vi "Lab Panel V5.23.vi"() -> ()   [LabVIEW 2013] (continued)
                          }
                        }
                        n2194 = local read "Panel #"() -> (w3891:dbl)
                        n2195 = case shown="1" w3891 {
                          tunnel: w3892 -> [_ w3899]
                          tunnel: w3889 -> [_ w3898]
                          frame 0, Default {
                          }
                          frame 1 {
                            n2196 = Multiply(x=w3899, y=w3898) -> (x*y=w3897:dbl)
                            n2197 = Subtract(x=w3897, y=272) -> (x-y=w3895:dbl)
                            "Amb Tp" <- w3895
                            n2198 = local write "Ref deg C"(w3895) -> ()
                          }
                        }
                        "deg C (volts)" <- w3889
                      }
                      frame True {
                      }
                    }
                  }
                }
              }
            }
          }
          frame #12 {
            # "save test data to file"
            n2199 = Get Date/Time In Seconds() -> (seconds since 1Jan1904=w3900:timestamp)
            "File Time Stamp" <- w3900
            n2200 = local read "on loops"() -> (w3919:dbl)
            n2201 = local read "jig cycle"() -> (w3916:dbl)
            n2202 = Format Date/Time String(time format string (%c)="%H:%M%:%S", seconds (now)=w3900) -> (date/time string=w3904:string)  [unwired: 1 in]
            n2203 = Add(x=w3919, y=2) -> (x+y=w3917:dbl)
            n2204 = Build Array(w3904) -> (w3903:string[])
            n2205 = Equal?(x=w3916, y=1) -> (x = y?=w3902:bool)
            n2206 = Equal?(x=w3916, y=w3917) -> (x = y?=w3901:bool)
            n2207 = stacked-sequence {
              tunnel: w3915 -> [w3925 _ _ _ _ _ _ _ _ _]
              tunnel: w3914 -> [_ w4001 _ _ _ _ _ _ _ _]
              tunnel: w3913 -> [_ _ w4081 _ _ _ _ _ _ _]
              tunnel: w3912 -> [_ _ _ w4161 _ _ _ _ _ _]
              tunnel: w3911 -> [_ _ _ _ w4241 _ _ _ _ _]
              tunnel: w3910 -> [_ _ _ _ _ w4321 _ _ _ _]
              tunnel: w3909 -> [_ _ _ _ _ _ w4401 _ _ _]
              tunnel: w3908 -> [_ _ _ _ _ _ _ w4481 _ _]
              tunnel: w3907 -> [_ _ _ _ _ _ _ _ w4561 _]
              tunnel: w3906 -> [_ _ _ _ _ _ _ _ _ w4641]
              tunnel: w3903 -> [w3924 w4005 w4085 w4165 w4245 w4325 w4405 w4485 w4565 w4645]
              tunnel: w3902 -> [w3923 w4004 w4084 w4164 w4244 w4324 w4404 w4484 w4564 w4644]
              tunnel: w3901 -> [w3922 w4003 w4083 w4163 w4243 w4323 w4403 w4483 w4563 w4643]
              tunnel: w3900 -> [w3921 w4002 w4082 w4162 w4242 w4322 w4402 w4482 w4562 w4642]
              frame #0 {
                n2208 = case shown="True" w3925 {
                  tunnel: w3924 -> [_ w3930]
                  tunnel: w3923 -> [_ w3929]
                  tunnel: w3922 -> [_ w3927]
                  tunnel: w3921 -> [_ w3926]
                  frame False {
                  }
                  frame True {
                    n2209 = local read "DISP LAB01-1"() -> (w3931:T4)
                    n2210 = local read "SIG LAB01-1"() -> (w3932:T2)
                    n2211 = local read "ON L01-1"() -> (w3928:cluster{"amps":dbl, "volts":dbl, "pf":dbl})
                    n2212 = Unbundle(w3932) -> ("AMPS"=w3938:dbl, "VOLTS"=w3936:dbl, "PF"=w3935:dbl, "Tmp Live"=w3934:dbl, "Tmp Neut"=w3937:dbl)
                    n2213 = Unbundle(w3931) -> ("CYCLE"=w3933:dbl)  [unwired: 2 out]
                    n2214 = stacked-sequence {
                      tunnel: w3938 -> [w3942 w3961]
                      tunnel: w3937 -> [_ w3960]
                      tunnel: w3936 -> [w3941 w3959]
                      tunnel: w3935 -> [w3940 w3958]
                      tunnel: w3934 -> [_ w3957]
                      tunnel: w3933 -> [_ w3956]
                      tunnel: w3930 -> [_ w3955]
                      tunnel: w3929 -> [w3943 _]
                      tunnel: w3928 -> [w3939 w3953]
                      tunnel: w3927 -> [_ w3954]
                      tunnel: w3926 -> [_ w3949]
                      frame #0 {
                        n2215 = case shown="True" w3943 {
                          tunnel: w3942 -> [_ w3948]
                          tunnel: w3941 -> [_ w3947]
                          tunnel: w3940 -> [_ w3946]
                          tunnel: w3939 -> [_ w3944]
                          frame False {
                          }
                          frame True {
                            n2216 = Bundle(cluster=w3944, "amps"=w3948, "volts"=w3947, "pf"=w3946) -> (w3945:cluster{"amps":dbl, "volts":dbl, "pf":dbl})
                            n2217 = local write "ON L01-1"(w3945) -> ()
                          }
                        }
                      }
                      frame #1 {
                        n2218 = Unbundle(w3953) -> ("amps"=w3952:dbl, "volts"=w3951:dbl, "pf"=w3950:dbl)
                        n2219 = case shown="True" w3954 {
                          tunnel: w3961 -> [_ w3962]
                          tunnel: w3960 -> [_ w4000]
                          tunnel: w3959 -> [_ _]
                          tunnel: w3958 -> [_ _]
                          tunnel: w3957 -> [_ w3999]
                          tunnel: w3956 -> [_ w3998]
                          tunnel: w3955 -> [_ w3966]
                          tunnel: w3952 -> [_ w3963]
                          tunnel: w3951 -> [_ w3995]
                          tunnel: w3950 -> [_ w3994]
                          tunnel: w3949 -> [_ w3964]
                          frame False {
                          }
                          frame True {
                            n2220 = local read "TDMS LAB01-1"() -> (w3997:refnum<k34>)
                            n2221 = Build Array(w3995) -> (w3991:dbl[])
                            n2222 = Build Array(w3994) -> (w3990:dbl[])
                            n2223 = Build Array(w3999) -> (w3989:dbl[])
                            n2224 = Build Array(w4000) -> (w3988:dbl[])
                            n2225 = Build Array(w3963) -> (w3993:dbl[])
                            n2226 = Build Array(w3962) -> (w3992:dbl[])
                            n2227 = Build Array(w3998) -> (w3987:dbl[])
                            n2228 = Build Array("AMPS ON", "AMPS OFF", "VOLTS", "PF", "TEMP Live", "TEMP Neut", "CYCLE") -> (w3971:string[])
                            n2229 = Bundle By Name("Y"=w3993, "t0"=w3964) -> (w3986:waveform(dbl))  [unwired: 1 in]
                            n2230 = Bundle By Name("Y"=w3992, "t0"=w3964) -> (w3985:waveform(dbl))  [unwired: 1 in]
                            n2231 = Bundle By Name("Y"=w3991, "t0"=w3964) -> (w3984:waveform(dbl))  [unwired: 1 in]
                            n2232 = Bundle By Name("Y"=w3990, "t0"=w3964) -> (w3983:waveform(dbl))  [unwired: 1 in]
                            n2233 = Bundle By Name("Y"=w3989, "t0"=w3964) -> (w3982:waveform(dbl))  [unwired: 1 in]
                            n2234 = Bundle By Name("Y"=w3988, "t0"=w3964) -> (w3981:waveform(dbl))  [unwired: 1 in]
                            n2235 = Bundle By Name("Y"=w3987, "t0"=w3964) -> (w3980:waveform(dbl))  [unwired: 1 in]
                            n2236 = Build Array(w3986, w3985, w3984, w3983, w3982, w3981, w3980) -> (w3979:waveform(dbl)[])
                            n2237 = TDMS Write(0:w3997, 5:"TEST VALUES", 7:w3971, 9:w3979) -> (4:w3970:refnum<k34>, 6:w3969:string, 15:w3968:errorcluster)  [unwired: 2 in, 1 out]
                            n2238 = TDMS Write(0:w3970, 5:w3969, 7:"TIME", 9:w3966, 11:w3968) -> (15:w3965:errorcluster)  [unwired: 1 in, 3 out]
                            n2239 = local write "data file error"(w3965) -> ()
                          }
                        }
                      }
                    }
                  }
                }
              }
              frame #1 {
                n2240 = case shown="True" w4001 {
                  tunnel: w4005 -> [_ w4010]
                  tunnel: w4004 -> [_ w4009]
                  tunnel: w4003 -> [_ w4007]
                  tunnel: w4002 -> [_ w4006]
                  frame False {
                  }
                  frame True {
                    n2241 = local read "DISP LAB01-2"() -> (w4011:T4)
                    n2242 = local read "SIG LAB01-2"() -> (w4012:T2)
                    n2243 = local read "ON L01-2"() -> (w4008:cluster{"amps":dbl, "volts":dbl, "pf":dbl})
                    n2244 = Unbundle(w4012) -> ("AMPS"=w4018:dbl, "VOLTS"=w4016:dbl, "PF"=w4015:dbl, "Tmp Live"=w4014:dbl, "Tmp Neut"=w4017:dbl)
                    n2245 = Unbundle(w4011) -> ("CYCLE"=w4013:dbl)  [unwired: 2 out]
                    n2246 = stacked-sequence {
                      tunnel: w4018 -> [w4022 w4041]
                      tunnel: w4017 -> [_ w4040]
                      tunnel: w4016 -> [w4021 w4039]
                      tunnel: w4015 -> [w4020 w4038]
                      tunnel: w4014 -> [_ w4037]
                      tunnel: w4013 -> [_ w4036]
                      tunnel: w4010 -> [_ w4035]
                      tunnel: w4009 -> [w4023 _]
                      tunnel: w4008 -> [w4019 w4033]
                      tunnel: w4007 -> [_ w4034]
                      tunnel: w4006 -> [_ w4029]
                      frame #0 {
                        n2247 = case shown="True" w4023 {
                          tunnel: w4022 -> [_ w4028]
                          tunnel: w4021 -> [_ w4027]
                          tunnel: w4020 -> [_ w4026]
                          tunnel: w4019 -> [_ w4024]
                          frame False {
                          }
                          frame True {
                            n2248 = Bundle(cluster=w4024, "amps"=w4028, "volts"=w4027, "pf"=w4026) -> (w4025:cluster{"amps":dbl, "volts":dbl, "pf":dbl})
                            n2249 = local write "ON L01-2"(w4025) -> ()
                          }
                        }
                      }
                      frame #1 {
                        n2250 = Unbundle(w4033) -> ("amps"=w4032:dbl, "volts"=w4031:dbl, "pf"=w4030:dbl)
                        n2251 = case shown="True" w4034 {
                          tunnel: w4041 -> [_ w4073]
                          tunnel: w4040 -> [_ w4080]
                          tunnel: w4039 -> [_ _]
                          tunnel: w4038 -> [_ _]
                          tunnel: w4037 -> [_ w4079]
                          tunnel: w4036 -> [_ w4078]
                          tunnel: w4035 -> [_ w4043]
                          tunnel: w4032 -> [_ w4075]
                          tunnel: w4031 -> [_ w4074]
                          tunnel: w4030 -> [_ w4072]
                          tunnel: w4029 -> [_ w4064]
                          frame False {
                          }
                          frame True {
                            n2252 = local read "TDMS LAB01-2"() -> (w4077:refnum<k34>)
                            n2253 = Build Array(w4074) -> (w4069:dbl[])
                            n2254 = Build Array(w4072) -> (w4068:dbl[])
                            n2255 = Build Array(w4079) -> (w4067:dbl[])
                            n2256 = Build Array(w4080) -> (w4066:dbl[])
                            n2257 = Build Array(w4075) -> (w4071:dbl[])
                            n2258 = Build Array(w4073) -> (w4070:dbl[])
                            n2259 = Build Array(w4078) -> (w4065:dbl[])
                            n2260 = Build Array("AMPS ON", "AMPS OFF", "VOLTS", "PF", "TEMP Live", "TEMP Neut", "CYCLE") -> (w4048:string[])
                            n2261 = Bundle By Name("Y"=w4071, "t0"=w4064) -> (w4063:waveform(dbl))  [unwired: 1 in]
                            n2262 = Bundle By Name("Y"=w4070, "t0"=w4064) -> (w4062:waveform(dbl))  [unwired: 1 in]
                            n2263 = Bundle By Name("Y"=w4069, "t0"=w4064) -> (w4061:waveform(dbl))  [unwired: 1 in]
                            n2264 = Bundle By Name("Y"=w4068, "t0"=w4064) -> (w4060:waveform(dbl))  [unwired: 1 in]
                            n2265 = Bundle By Name("Y"=w4067, "t0"=w4064) -> (w4059:waveform(dbl))  [unwired: 1 in]
                            n2266 = Bundle By Name("Y"=w4066, "t0"=w4064) -> (w4058:waveform(dbl))  [unwired: 1 in]
                            n2267 = Bundle By Name("Y"=w4065, "t0"=w4064) -> (w4057:waveform(dbl))  [unwired: 1 in]
                            n2268 = Build Array(w4063, w4062, w4061, w4060, w4059, w4058, w4057) -> (w4056:waveform(dbl)[])
                            n2269 = TDMS Write(0:w4077, 5:"TEST VALUES", 7:w4048, 9:w4056) -> (4:w4047:refnum<k34>, 6:w4046:string, 15:w4045:errorcluster)  [unwired: 2 in, 1 out]
                            n2270 = TDMS Write(0:w4047, 5:w4046, 7:"TIME", 9:w4043, 11:w4045) -> (15:w4042:errorcluster)  [unwired: 1 in, 3 out]
                            n2271 = local write "data file error"(w4042) -> ()
                          }
                        }
                      }
                    }
                  }
                }
              }
              frame #2 {
                n2272 = case shown="True" w4081 {
                  tunnel: w4085 -> [_ w4090]
                  tunnel: w4084 -> [_ w4089]
                  tunnel: w4083 -> [_ w4087]
                  tunnel: w4082 -> [_ w4086]
                  frame False {
                  }
                  frame True {
                    n2273 = local read "DISP LAB02-1"() -> (w4091:T4)
                    n2274 = local read "SIG LAB02-1"() -> (w4092:T2)
                    n2275 = local read "ON L02-1"() -> (w4088:cluster{"amps":dbl, "volts":dbl, "pf":dbl})
                    n2276 = Unbundle(w4092) -> ("AMPS"=w4098:dbl, "VOLTS"=w4096:dbl, "PF"=w4095:dbl, "Tmp Live"=w4094:dbl, "Tmp Neut"=w4097:dbl)
                    n2277 = Unbundle(w4091) -> ("CYCLE"=w4093:dbl)  [unwired: 2 out]
                    n2278 = stacked-sequence {
                      tunnel: w4098 -> [w4102 w4121]
                      tunnel: w4097 -> [_ w4120]
                      tunnel: w4096 -> [w4101 w4119]
                      tunnel: w4095 -> [w4100 w4118]
                      tunnel: w4094 -> [_ w4117]
                      tunnel: w4093 -> [_ w4116]
                      tunnel: w4090 -> [_ w4115]
                      tunnel: w4089 -> [w4103 _]
                      tunnel: w4088 -> [w4099 w4113]
                      tunnel: w4087 -> [_ w4114]
                      tunnel: w4086 -> [_ w4109]
                      frame #0 {
                        n2279 = case shown="True" w4103 {
                          tunnel: w4102 -> [_ w4108]
                          tunnel: w4101 -> [_ w4107]
                          tunnel: w4100 -> [_ w4106]
                          tunnel: w4099 -> [_ w4104]
                          frame False {
                          }
                          frame True {
                            n2280 = Bundle(cluster=w4104, "amps"=w4108, "volts"=w4107, "pf"=w4106) -> (w4105:cluster{"amps":dbl, "volts":dbl, "pf":dbl})
                            n2281 = local write "ON L02-1"(w4105) -> ()
                          }
                        }
                      }
                      frame #1 {
                        n2282 = Unbundle(w4113) -> ("amps"=w4112:dbl, "volts"=w4111:dbl, "pf"=w4110:dbl)
                        n2283 = case shown="True" w4114 {
                          tunnel: w4121 -> [_ w4153]
                          tunnel: w4120 -> [_ w4160]
                          tunnel: w4119 -> [_ _]
                          tunnel: w4118 -> [_ _]
                          tunnel: w4117 -> [_ w4159]
                          tunnel: w4116 -> [_ w4158]
                          tunnel: w4115 -> [_ w4123]
                          tunnel: w4112 -> [_ w4155]
                          tunnel: w4111 -> [_ w4154]
                          tunnel: w4110 -> [_ w4152]
                          tunnel: w4109 -> [_ w4144]
                          frame False {
                          }
                          frame True {
                            n2284 = local read "TDMS LAB02-1"() -> (w4157:refnum<k34>)
                            n2285 = Build Array(w4154) -> (w4149:dbl[])
                            n2286 = Build Array(w4152) -> (w4148:dbl[])
                            n2287 = Build Array(w4159) -> (w4147:dbl[])
                            n2288 = Build Array(w4160) -> (w4146:dbl[])
                            n2289 = Build Array(w4155) -> (w4151:dbl[])
                            n2290 = Build Array(w4153) -> (w4150:dbl[])
                            n2291 = Build Array(w4158) -> (w4145:dbl[])
                            n2292 = Build Array("AMPS ON", "AMPS OFF", "VOLTS", "PF", "TEMP Live", "TEMP Neut", "CYCLE") -> (w4128:string[])
                            n2293 = Bundle By Name("Y"=w4151, "t0"=w4144) -> (w4143:waveform(dbl))  [unwired: 1 in]
                            n2294 = Bundle By Name("Y"=w4150, "t0"=w4144) -> (w4142:waveform(dbl))  [unwired: 1 in]
                            n2295 = Bundle By Name("Y"=w4149, "t0"=w4144) -> (w4141:waveform(dbl))  [unwired: 1 in]
                            n2296 = Bundle By Name("Y"=w4148, "t0"=w4144) -> (w4140:waveform(dbl))  [unwired: 1 in]
                            n2297 = Bundle By Name("Y"=w4147, "t0"=w4144) -> (w4139:waveform(dbl))  [unwired: 1 in]
                            n2298 = Bundle By Name("Y"=w4146, "t0"=w4144) -> (w4138:waveform(dbl))  [unwired: 1 in]
                            n2299 = Bundle By Name("Y"=w4145, "t0"=w4144) -> (w4137:waveform(dbl))  [unwired: 1 in]
                            n2300 = Build Array(w4143, w4142, w4141, w4140, w4139, w4138, w4137) -> (w4136:waveform(dbl)[])
                            n2301 = TDMS Write(0:w4157, 5:"TEST VALUES", 7:w4128, 9:w4136) -> (4:w4127:refnum<k34>, 6:w4126:string, 15:w4125:errorcluster)  [unwired: 2 in, 1 out]
                            n2302 = TDMS Write(0:w4127, 5:w4126, 7:"TIME", 9:w4123, 11:w4125) -> (15:w4122:errorcluster)  [unwired: 1 in, 3 out]
                            n2303 = local write "data file error"(w4122) -> ()
                          }
                        }
                      }
                    }
                  }
                }
              }
              frame #3 {
                n2304 = case shown="True" w4161 {
                  tunnel: w4165 -> [_ w4170]
                  tunnel: w4164 -> [_ w4169]
                  tunnel: w4163 -> [_ w4167]
                  tunnel: w4162 -> [_ w4166]
                  frame False {
                  }
                  frame True {
                    n2305 = local read "DISP LAB02-2"() -> (w4171:T4)
                    n2306 = local read "SIG LAB02-2"() -> (w4172:T2)
                    n2307 = local read "ON L02-2"() -> (w4168:cluster{"amps":dbl, "volts":dbl, "pf":dbl})
                    n2308 = Unbundle(w4172) -> ("AMPS"=w4178:dbl, "VOLTS"=w4176:dbl, "PF"=w4175:dbl, "Tmp Live"=w4174:dbl, "Tmp Neut"=w4177:dbl)
                    n2309 = Unbundle(w4171) -> ("CYCLE"=w4173:dbl)  [unwired: 2 out]
                    n2310 = stacked-sequence {
                      tunnel: w4178 -> [w4182 w4201]
                      tunnel: w4177 -> [_ w4200]
                      tunnel: w4176 -> [w4181 w4199]
                      tunnel: w4175 -> [w4180 w4198]
                      tunnel: w4174 -> [_ w4197]
                      tunnel: w4173 -> [_ w4196]
                      tunnel: w4170 -> [_ w4195]
                      tunnel: w4169 -> [w4183 _]
                      tunnel: w4168 -> [w4179 w4193]
                      tunnel: w4167 -> [_ w4194]
                      tunnel: w4166 -> [_ w4189]
                      frame #0 {
                        n2311 = case shown="True" w4183 {
                          tunnel: w4182 -> [_ w4188]
                          tunnel: w4181 -> [_ w4187]
                          tunnel: w4180 -> [_ w4186]
                          tunnel: w4179 -> [_ w4184]
                          frame False {
                          }
                          frame True {
                            n2312 = Bundle(cluster=w4184, "amps"=w4188, "volts"=w4187, "pf"=w4186) -> (w4185:cluster{"amps":dbl, "volts":dbl, "pf":dbl})
                            n2313 = local write "ON L02-2"(w4185) -> ()
                          }
                        }
                      }
                      frame #1 {
                        n2314 = Unbundle(w4193) -> ("amps"=w4192:dbl, "volts"=w4191:dbl, "pf"=w4190:dbl)
                        n2315 = case shown="True" w4194 {
                          tunnel: w4201 -> [_ w4233]
                          tunnel: w4200 -> [_ w4240]
                          tunnel: w4199 -> [_ _]
                          tunnel: w4198 -> [_ _]
                          tunnel: w4197 -> [_ w4239]
                          tunnel: w4196 -> [_ w4238]
                          tunnel: w4195 -> [_ w4203]
                          tunnel: w4192 -> [_ w4235]
                          tunnel: w4191 -> [_ w4234]
                          tunnel: w4190 -> [_ w4232]
                          tunnel: w4189 -> [_ w4224]
                          frame False {
                          }
                          frame True {
                            n2316 = local read "TDMS LAB02-2"() -> (w4237:refnum<k34>)
                            n2317 = Build Array(w4234) -> (w4229:dbl[])
                            n2318 = Build Array(w4232) -> (w4228:dbl[])
                            n2319 = Build Array(w4239) -> (w4227:dbl[])
                            n2320 = Build Array(w4240) -> (w4226:dbl[])
                            n2321 = Build Array(w4235) -> (w4231:dbl[])
                            n2322 = Build Array(w4233) -> (w4230:dbl[])
                            n2323 = Build Array(w4238) -> (w4225:dbl[])
                            n2324 = Build Array("AMPS ON", "AMPS OFF", "VOLTS", "PF", "TEMP Live", "TEMP Neut", "CYCLE") -> (w4208:string[])
                            n2325 = Bundle By Name("Y"=w4231, "t0"=w4224) -> (w4223:waveform(dbl))  [unwired: 1 in]
                            n2326 = Bundle By Name("Y"=w4230, "t0"=w4224) -> (w4222:waveform(dbl))  [unwired: 1 in]
                            n2327 = Bundle By Name("Y"=w4229, "t0"=w4224) -> (w4221:waveform(dbl))  [unwired: 1 in]
                            n2328 = Bundle By Name("Y"=w4228, "t0"=w4224) -> (w4220:waveform(dbl))  [unwired: 1 in]
                            n2329 = Bundle By Name("Y"=w4227, "t0"=w4224) -> (w4219:waveform(dbl))  [unwired: 1 in]
                            n2330 = Bundle By Name("Y"=w4226, "t0"=w4224) -> (w4218:waveform(dbl))  [unwired: 1 in]
                            n2331 = Bundle By Name("Y"=w4225, "t0"=w4224) -> (w4217:waveform(dbl))  [unwired: 1 in]
                            n2332 = Build Array(w4223, w4222, w4221, w4220, w4219, w4218, w4217) -> (w4216:waveform(dbl)[])
                            n2333 = TDMS Write(0:w4237, 5:"TEST VALUES", 7:w4208, 9:w4216) -> (4:w4207:refnum<k34>, 6:w4206:string, 15:w4205:errorcluster)  [unwired: 2 in, 1 out]
                            n2334 = TDMS Write(0:w4207, 5:w4206, 7:"TIME", 9:w4203, 11:w4205) -> (15:w4202:errorcluster)  [unwired: 1 in, 3 out]
                            n2335 = local write "data file error"(w4202) -> ()
                          }
                        }
                      }
                    }
                  }
                }
              }
              frame #4 {
                n2336 = case shown="True" w4241 {
                  tunnel: w4245 -> [_ w4250]
                  tunnel: w4244 -> [_ w4249]
                  tunnel: w4243 -> [_ w4247]
                  tunnel: w4242 -> [_ w4246]
                  frame False {
                  }
                  frame True {
                    n2337 = local read "DISP LAB03-1"() -> (w4251:T4)
                    n2338 = local read "SIG LAB03-1"() -> (w4252:T2)
                    n2339 = local read "ON L03-1"() -> (w4248:cluster{"amps":dbl, "volts":dbl, "pf":dbl})
                    n2340 = Unbundle(w4252) -> ("AMPS"=w4258:dbl, "VOLTS"=w4256:dbl, "PF"=w4255:dbl, "Tmp Live"=w4254:dbl, "Tmp Neut"=w4257:dbl)
                    n2341 = Unbundle(w4251) -> ("CYCLE"=w4253:dbl)  [unwired: 2 out]
                    n2342 = stacked-sequence {
                      tunnel: w4258 -> [w4262 w4281]
                      tunnel: w4257 -> [_ w4280]
                      tunnel: w4256 -> [w4261 w4279]
                      tunnel: w4255 -> [w4260 w4278]
                      tunnel: w4254 -> [_ w4277]
                      tunnel: w4253 -> [_ w4276]
                      tunnel: w4250 -> [_ w4275]
                      tunnel: w4249 -> [w4263 _]
                      tunnel: w4248 -> [w4259 w4273]
                      tunnel: w4247 -> [_ w4274]
                      tunnel: w4246 -> [_ w4269]
                      frame #0 {
                        n2343 = case shown="True" w4263 {
                          tunnel: w4262 -> [_ w4268]
                          tunnel: w4261 -> [_ w4267]
                          tunnel: w4260 -> [_ w4266]
                          tunnel: w4259 -> [_ w4264]
                          frame False {
                          }
                          frame True {
                            n2344 = Bundle(cluster=w4264, "amps"=w4268, "volts"=w4267, "pf"=w4266) -> (w4265:cluster{"amps":dbl, "volts":dbl, "pf":dbl})
                            n2345 = local write "ON L03-1"(w4265) -> ()
                          }
                        }
                      }
                      frame #1 {
                        n2346 = Unbundle(w4273) -> ("amps"=w4272:dbl, "volts"=w4271:dbl, "pf"=w4270:dbl)
                        n2347 = case shown="True" w4274 {
                          tunnel: w4281 -> [_ w4313]
                          tunnel: w4280 -> [_ w4320]
                          tunnel: w4279 -> [_ _]
                          tunnel: w4278 -> [_ _]
                          tunnel: w4277 -> [_ w4319]
                          tunnel: w4276 -> [_ w4318]
                          tunnel: w4275 -> [_ w4283]
                          tunnel: w4272 -> [_ w4315]
                          tunnel: w4271 -> [_ w4314]
                          tunnel: w4270 -> [_ w4312]
                          tunnel: w4269 -> [_ w4304]
                          frame False {
                          }
                          frame True {
                            n2348 = local read "TDMS LAB03-1"() -> (w4317:refnum<k34>)
                            n2349 = Build Array(w4314) -> (w4309:dbl[])
                            n2350 = Build Array(w4312) -> (w4308:dbl[])
                            n2351 = Build Array(w4319) -> (w4307:dbl[])
                            n2352 = Build Array(w4320) -> (w4306:dbl[])
                            n2353 = Build Array(w4315) -> (w4311:dbl[])
                            n2354 = Build Array(w4313) -> (w4310:dbl[])
                            n2355 = Build Array(w4318) -> (w4305:dbl[])
                            n2356 = Build Array("AMPS ON", "AMPS OFF", "VOLTS", "PF", "TEMP Live", "TEMP Neut", "CYCLE") -> (w4288:string[])
                            n2357 = Bundle By Name("Y"=w4311, "t0"=w4304) -> (w4303:waveform(dbl))  [unwired: 1 in]
                            n2358 = Bundle By Name("Y"=w4310, "t0"=w4304) -> (w4302:waveform(dbl))  [unwired: 1 in]
                            n2359 = Bundle By Name("Y"=w4309, "t0"=w4304) -> (w4301:waveform(dbl))  [unwired: 1 in]
                            n2360 = Bundle By Name("Y"=w4308, "t0"=w4304) -> (w4300:waveform(dbl))  [unwired: 1 in]
                            n2361 = Bundle By Name("Y"=w4307, "t0"=w4304) -> (w4299:waveform(dbl))  [unwired: 1 in]
                            n2362 = Bundle By Name("Y"=w4306, "t0"=w4304) -> (w4298:waveform(dbl))  [unwired: 1 in]
                            n2363 = Bundle By Name("Y"=w4305, "t0"=w4304) -> (w4297:waveform(dbl))  [unwired: 1 in]
                            n2364 = Build Array(w4303, w4302, w4301, w4300, w4299, w4298, w4297) -> (w4296:waveform(dbl)[])
                            n2365 = TDMS Write(0:w4317, 5:"TEST VALUES", 7:w4288, 9:w4296) -> (4:w4287:refnum<k34>, 6:w4286:string, 15:w4285:errorcluster)  [unwired: 2 in, 1 out]
                            n2366 = TDMS Write(0:w4287, 5:w4286, 7:"TIME", 9:w4283, 11:w4285) -> (15:w4282:errorcluster)  [unwired: 1 in, 3 out]
                            n2367 = local write "data file error"(w4282) -> ()
                          }
                        }
                      }
                    }
                  }
                }
              }
              frame #5 {
                n2368 = case shown="True" w4321 {
                  tunnel: w4325 -> [_ w4330]
                  tunnel: w4324 -> [_ w4329]
                  tunnel: w4323 -> [_ w4327]
                  tunnel: w4322 -> [_ w4326]
                  frame False {
                  }
                  frame True {
                    n2369 = local read "DISP LAB03-2"() -> (w4331:T4)
                    n2370 = local read "SIG LAB03-2"() -> (w4332:T2)
                    n2371 = local read "ON L03-2"() -> (w4328:cluster{"amps":dbl, "volts":dbl, "pf":dbl})
                    n2372 = Unbundle(w4332) -> ("AMPS"=w4338:dbl, "VOLTS"=w4336:dbl, "PF"=w4335:dbl, "Tmp Live"=w4334:dbl, "Tmp Neut"=w4337:dbl)
                    n2373 = Unbundle(w4331) -> ("CYCLE"=w4333:dbl)  [unwired: 2 out]
                    n2374 = stacked-sequence {
                      tunnel: w4338 -> [w4342 w4361]
                      tunnel: w4337 -> [_ w4360]
                      tunnel: w4336 -> [w4341 w4359]
                      tunnel: w4335 -> [w4340 w4358]
                      tunnel: w4334 -> [_ w4357]
                      tunnel: w4333 -> [_ w4356]
                      tunnel: w4330 -> [_ w4355]
                      tunnel: w4329 -> [w4343 _]
                      tunnel: w4328 -> [w4339 w4353]
                      tunnel: w4327 -> [_ w4354]
                      tunnel: w4326 -> [_ w4349]
                      frame #0 {
                        n2375 = case shown="True" w4343 {
                          tunnel: w4342 -> [_ w4348]
                          tunnel: w4341 -> [_ w4347]
                          tunnel: w4340 -> [_ w4346]
                          tunnel: w4339 -> [_ w4344]
                          frame False {
                          }
                          frame True {
                            n2376 = Bundle(cluster=w4344, "amps"=w4348, "volts"=w4347, "pf"=w4346) -> (w4345:cluster{"amps":dbl, "volts":dbl, "pf":dbl})
                            n2377 = local write "ON L03-2"(w4345) -> ()
                          }
                        }
                      }
                      frame #1 {
                        n2378 = Unbundle(w4353) -> ("amps"=w4352:dbl, "volts"=w4351:dbl, "pf"=w4350:dbl)
                        n2379 = case shown="True" w4354 {
                          tunnel: w4361 -> [_ w4393]
                          tunnel: w4360 -> [_ w4400]
                          tunnel: w4359 -> [_ _]
                          tunnel: w4358 -> [_ _]
                          tunnel: w4357 -> [_ w4399]
                          tunnel: w4356 -> [_ w4398]
                          tunnel: w4355 -> [_ w4363]
                          tunnel: w4352 -> [_ w4395]
                          tunnel: w4351 -> [_ w4394]
                          tunnel: w4350 -> [_ w4392]
                          tunnel: w4349 -> [_ w4384]
                          frame False {
                          }
                          frame True {
                            n2380 = local read "TDMS LAB03-2"() -> (w4397:refnum<k34>)
                            n2381 = Build Array(w4394) -> (w4389:dbl[])
                            n2382 = Build Array(w4392) -> (w4388:dbl[])
                            n2383 = Build Array(w4399) -> (w4387:dbl[])
                            n2384 = Build Array(w4400) -> (w4386:dbl[])
                            n2385 = Build Array(w4395) -> (w4391:dbl[])
                            n2386 = Build Array(w4393) -> (w4390:dbl[])
                            n2387 = Build Array(w4398) -> (w4385:dbl[])
                            n2388 = Build Array("AMPS ON", "AMPS OFF", "VOLTS", "PF", "TEMP Live", "TEMP Neut", "CYCLE") -> (w4368:string[])
                            n2389 = Bundle By Name("Y"=w4391, "t0"=w4384) -> (w4383:waveform(dbl))  [unwired: 1 in]
                            n2390 = Bundle By Name("Y"=w4390, "t0"=w4384) -> (w4382:waveform(dbl))  [unwired: 1 in]
                            n2391 = Bundle By Name("Y"=w4389, "t0"=w4384) -> (w4381:waveform(dbl))  [unwired: 1 in]
                            n2392 = Bundle By Name("Y"=w4388, "t0"=w4384) -> (w4380:waveform(dbl))  [unwired: 1 in]
                            n2393 = Bundle By Name("Y"=w4387, "t0"=w4384) -> (w4379:waveform(dbl))  [unwired: 1 in]
                            n2394 = Bundle By Name("Y"=w4386, "t0"=w4384) -> (w4378:waveform(dbl))  [unwired: 1 in]
                            n2395 = Bundle By Name("Y"=w4385, "t0"=w4384) -> (w4377:waveform(dbl))  [unwired: 1 in]
                            n2396 = Build Array(w4383, w4382, w4381, w4380, w4379, w4378, w4377) -> (w4376:waveform(dbl)[])
                            n2397 = TDMS Write(0:w4397, 5:"TEST VALUES", 7:w4368, 9:w4376) -> (4:w4367:refnum<k34>, 6:w4366:string, 15:w4365:errorcluster)  [unwired: 2 in, 1 out]
                            n2398 = TDMS Write(0:w4367, 5:w4366, 7:"TIME", 9:w4363, 11:w4365) -> (15:w4362:errorcluster)  [unwired: 1 in, 3 out]
                            n2399 = local write "data file error"(w4362) -> ()
                          }
                        }
                      }
                    }
                  }
                }
              }
              frame #6 {
                n2400 = case shown="True" w4401 {
                  tunnel: w4405 -> [_ w4410]
                  tunnel: w4404 -> [_ w4409]
                  tunnel: w4403 -> [_ w4407]
                  tunnel: w4402 -> [_ w4406]
                  frame False {
                  }
                  frame True {
                    n2401 = local read "DISP LAB04-1"() -> (w4411:T4)
                    n2402 = local read "SIG LAB04-1"() -> (w4412:T2)
                    n2403 = local read "ON L04-1"() -> (w4408:cluster{"amps":dbl, "volts":dbl, "pf":dbl})
                    n2404 = Unbundle(w4412) -> ("AMPS"=w4418:dbl, "VOLTS"=w4416:dbl, "PF"=w4415:dbl, "Tmp Live"=w4414:dbl, "Tmp Neut"=w4417:dbl)
                    n2405 = Unbundle(w4411) -> ("CYCLE"=w4413:dbl)  [unwired: 2 out]
                    n2406 = stacked-sequence {
                      tunnel: w4418 -> [w4422 w4441]
                      tunnel: w4417 -> [_ w4440]
                      tunnel: w4416 -> [w4421 w4439]
                      tunnel: w4415 -> [w4420 w4438]
                      tunnel: w4414 -> [_ w4437]
                      tunnel: w4413 -> [_ w4436]
                      tunnel: w4410 -> [_ w4435]
                      tunnel: w4409 -> [w4423 _]
                      tunnel: w4408 -> [w4419 w4433]
                      tunnel: w4407 -> [_ w4434]
                      tunnel: w4406 -> [_ w4429]
                      frame #0 {
                        n2407 = case shown="True" w4423 {
                          tunnel: w4422 -> [_ w4428]
                          tunnel: w4421 -> [_ w4427]
                          tunnel: w4420 -> [_ w4426]
                          tunnel: w4419 -> [_ w4424]
                          frame False {
                          }
                          frame True {
                            n2408 = Bundle(cluster=w4424, "amps"=w4428, "volts"=w4427, "pf"=w4426) -> (w4425:cluster{"amps":dbl, "volts":dbl, "pf":dbl})
                            n2409 = local write "ON L04-1"(w4425) -> ()
                          }
                        }
                      }
                      frame #1 {
                        n2410 = Unbundle(w4433) -> ("amps"=w4432:dbl, "volts"=w4431:dbl, "pf"=w4430:dbl)
                        n2411 = case shown="True" w4434 {
                          tunnel: w4441 -> [_ w4473]
                          tunnel: w4440 -> [_ w4480]
                          tunnel: w4439 -> [_ _]
                          tunnel: w4438 -> [_ _]
                          tunnel: w4437 -> [_ w4479]
                          tunnel: w4436 -> [_ w4478]
                          tunnel: w4435 -> [_ w4443]
                          tunnel: w4432 -> [_ w4475]
                          tunnel: w4431 -> [_ w4474]
                          tunnel: w4430 -> [_ w4472]
                          tunnel: w4429 -> [_ w4464]
                          frame False {
                          }
                          frame True {
                            n2412 = local read "TDMS LAB04-1"() -> (w4477:refnum<k34>)
                            n2413 = Build Array(w4474) -> (w4469:dbl[])
                            n2414 = Build Array(w4472) -> (w4468:dbl[])
                            n2415 = Build Array(w4479) -> (w4467:dbl[])
                            n2416 = Build Array(w4480) -> (w4466:dbl[])
                            n2417 = Build Array(w4475) -> (w4471:dbl[])
                            n2418 = Build Array(w4473) -> (w4470:dbl[])
                            n2419 = Build Array(w4478) -> (w4465:dbl[])
                            n2420 = Build Array("AMPS ON", "AMPS OFF", "VOLTS", "PF", "TEMP Live", "TEMP Neut", "CYCLE") -> (w4448:string[])
                            n2421 = Bundle By Name("Y"=w4471, "t0"=w4464) -> (w4463:waveform(dbl))  [unwired: 1 in]
                            n2422 = Bundle By Name("Y"=w4470, "t0"=w4464) -> (w4462:waveform(dbl))  [unwired: 1 in]
                            n2423 = Bundle By Name("Y"=w4469, "t0"=w4464) -> (w4461:waveform(dbl))  [unwired: 1 in]
                            n2424 = Bundle By Name("Y"=w4468, "t0"=w4464) -> (w4460:waveform(dbl))  [unwired: 1 in]
                            n2425 = Bundle By Name("Y"=w4467, "t0"=w4464) -> (w4459:waveform(dbl))  [unwired: 1 in]
                            n2426 = Bundle By Name("Y"=w4466, "t0"=w4464) -> (w4458:waveform(dbl))  [unwired: 1 in]
                            n2427 = Bundle By Name("Y"=w4465, "t0"=w4464) -> (w4457:waveform(dbl))  [unwired: 1 in]
                            n2428 = Build Array(w4463, w4462, w4461, w4460, w4459, w4458, w4457) -> (w4456:waveform(dbl)[])
                            n2429 = TDMS Write(0:w4477, 5:"TEST VALUES", 7:w4448, 9:w4456) -> (4:w4447:refnum<k34>, 6:w4446:string, 15:w4445:errorcluster)  [unwired: 2 in, 1 out]
                            n2430 = TDMS Write(0:w4447, 5:w4446, 7:"TIME", 9:w4443, 11:w4445) -> (15:w4442:errorcluster)  [unwired: 1 in, 3 out]
                            n2431 = local write "data file error"(w4442) -> ()
                          }
                        }
                      }
                    }
                  }
                }
              }
              frame #7 {
                n2432 = case shown="True" w4481 {
                  tunnel: w4485 -> [_ w4490]
                  tunnel: w4484 -> [_ w4489]
                  tunnel: w4483 -> [_ w4487]
                  tunnel: w4482 -> [_ w4486]
                  frame False {
                  }
                  frame True {
                    n2433 = local read "DISP LAB04-2"() -> (w4491:T4)
                    n2434 = local read "SIG LAB04-2"() -> (w4492:T2)
                    n2435 = local read "ON L04-2"() -> (w4488:cluster{"amps":dbl, "volts":dbl, "pf":dbl})
                    n2436 = Unbundle(w4492) -> ("AMPS"=w4498:dbl, "VOLTS"=w4496:dbl, "PF"=w4495:dbl, "Tmp Live"=w4494:dbl, "Tmp Neut"=w4497:dbl)
                    n2437 = Unbundle(w4491) -> ("CYCLE"=w4493:dbl)  [unwired: 2 out]
                    n2438 = stacked-sequence {
                      tunnel: w4498 -> [w4502 w4521]
                      tunnel: w4497 -> [_ w4520]
                      tunnel: w4496 -> [w4501 w4519]
                      tunnel: w4495 -> [w4500 w4518]
                      tunnel: w4494 -> [_ w4517]
                      tunnel: w4493 -> [_ w4516]
                      tunnel: w4490 -> [_ w4515]
                      tunnel: w4489 -> [w4503 _]
                      tunnel: w4488 -> [w4499 w4513]
                      tunnel: w4487 -> [_ w4514]
                      tunnel: w4486 -> [_ w4509]
                      frame #0 {
                        n2439 = case shown="True" w4503 {
                          tunnel: w4502 -> [_ w4508]
                          tunnel: w4501 -> [_ w4507]
                          tunnel: w4500 -> [_ w4506]
                          tunnel: w4499 -> [_ w4504]
                          frame False {
                          }
                          frame True {
                            n2440 = Bundle(cluster=w4504, "amps"=w4508, "volts"=w4507, "pf"=w4506) -> (w4505:cluster{"amps":dbl, "volts":dbl, "pf":dbl})
                            n2441 = local write "ON L04-2"(w4505) -> ()
                          }
                        }
                      }
                      frame #1 {
                        n2442 = Unbundle(w4513) -> ("amps"=w4512:dbl, "volts"=w4511:dbl, "pf"=w4510:dbl)
                        n2443 = case shown="True" w4514 {
                          tunnel: w4521 -> [_ w4553]
                          tunnel: w4520 -> [_ w4560]
                          tunnel: w4519 -> [_ _]
                          tunnel: w4518 -> [_ _]
                          tunnel: w4517 -> [_ w4559]
                          tunnel: w4516 -> [_ w4558]
                          tunnel: w4515 -> [_ w4523]
                          tunnel: w4512 -> [_ w4555]
                          tunnel: w4511 -> [_ w4554]
                          tunnel: w4510 -> [_ w4552]
                          tunnel: w4509 -> [_ w4544]
                          frame False {
                          }
                          frame True {
                            n2444 = local read "TDMS LAB04-2"() -> (w4557:refnum<k34>)
                            n2445 = Build Array(w4554) -> (w4549:dbl[])
                            n2446 = Build Array(w4552) -> (w4548:dbl[])
                            n2447 = Build Array(w4559) -> (w4547:dbl[])
                            n2448 = Build Array(w4560) -> (w4546:dbl[])
                            n2449 = Build Array(w4555) -> (w4551:dbl[])
                            n2450 = Build Array(w4553) -> (w4550:dbl[])
                            n2451 = Build Array(w4558) -> (w4545:dbl[])
                            n2452 = Build Array("AMPS ON", "AMPS OFF", "VOLTS", "PF", "TEMP Live", "TEMP Neut", "CYCLE") -> (w4528:string[])
                            n2453 = Bundle By Name("Y"=w4551, "t0"=w4544) -> (w4543:waveform(dbl))  [unwired: 1 in]
                            n2454 = Bundle By Name("Y"=w4550, "t0"=w4544) -> (w4542:waveform(dbl))  [unwired: 1 in]
                            n2455 = Bundle By Name("Y"=w4549, "t0"=w4544) -> (w4541:waveform(dbl))  [unwired: 1 in]
                            n2456 = Bundle By Name("Y"=w4548, "t0"=w4544) -> (w4540:waveform(dbl))  [unwired: 1 in]
                            n2457 = Bundle By Name("Y"=w4547, "t0"=w4544) -> (w4539:waveform(dbl))  [unwired: 1 in]
                            n2458 = Bundle By Name("Y"=w4546, "t0"=w4544) -> (w4538:waveform(dbl))  [unwired: 1 in]
                            n2459 = Bundle By Name("Y"=w4545, "t0"=w4544) -> (w4537:waveform(dbl))  [unwired: 1 in]
                            n2460 = Build Array(w4543, w4542, w4541, w4540, w4539, w4538, w4537) -> (w4536:waveform(dbl)[])
                            n2461 = TDMS Write(0:w4557, 5:"TEST VALUES", 7:w4528, 9:w4536) -> (4:w4527:refnum<k34>, 6:w4526:string, 15:w4525:errorcluster)  [unwired: 2 in, 1 out]
                            n2462 = TDMS Write(0:w4527, 5:w4526, 7:"TIME", 9:w4523, 11:w4525) -> (15:w4522:errorcluster)  [unwired: 1 in, 3 out]
                            n2463 = local write "data file error"(w4522) -> ()
                          }
                        }
                      }
                    }
                  }
                }
              }
              frame #8 {
                n2464 = case shown="True" w4561 {
                  tunnel: w4565 -> [_ w4570]
                  tunnel: w4564 -> [_ w4569]
                  tunnel: w4563 -> [_ w4567]
                  tunnel: w4562 -> [_ w4566]
                  frame False {
                  }
                  frame True {
                    n2465 = local read "DISP LAB05-1"() -> (w4571:T4)
                    n2466 = local read "SIG LAB05-1"() -> (w4572:T2)
                    n2467 = local read "ON L05-1"() -> (w4568:cluster{"amps":dbl, "volts":dbl, "pf":dbl})
                    n2468 = Unbundle(w4572) -> ("AMPS"=w4578:dbl, "VOLTS"=w4576:dbl, "PF"=w4575:dbl, "Tmp Live"=w4574:dbl, "Tmp Neut"=w4577:dbl)
                    n2469 = Unbundle(w4571) -> ("CYCLE"=w4573:dbl)  [unwired: 2 out]
                    n2470 = stacked-sequence {
                      tunnel: w4578 -> [w4582 w4601]
                      tunnel: w4577 -> [_ w4600]
                      tunnel: w4576 -> [w4581 w4599]
                      tunnel: w4575 -> [w4580 w4598]
                      tunnel: w4574 -> [_ w4597]
                      tunnel: w4573 -> [_ w4596]
                      tunnel: w4570 -> [_ w4595]
                      tunnel: w4569 -> [w4583 _]
                      tunnel: w4568 -> [w4579 w4593]
                      tunnel: w4567 -> [_ w4594]
                      tunnel: w4566 -> [_ w4589]
                      frame #0 {
                        n2471 = case shown="True" w4583 {
                          tunnel: w4582 -> [_ w4588]
                          tunnel: w4581 -> [_ w4587]
                          tunnel: w4580 -> [_ w4586]
                          tunnel: w4579 -> [_ w4584]
                          frame False {
                          }
                          frame True {
                            n2472 = Bundle(cluster=w4584, "amps"=w4588, "volts"=w4587, "pf"=w4586) -> (w4585:cluster{"amps":dbl, "volts":dbl, "pf":dbl})
                            n2473 = local write "ON L05-1"(w4585) -> ()
                          }
                        }
                      }
                      frame #1 {
                        n2474 = Unbundle(w4593) -> ("amps"=w4592:dbl, "volts"=w4591:dbl, "pf"=w4590:dbl)
                        n2475 = case shown="True" w4594 {
                          tunnel: w4601 -> [_ w4633]
                          tunnel: w4600 -> [_ w4640]
                          tunnel: w4599 -> [_ _]
                          tunnel: w4598 -> [_ _]
                          tunnel: w4597 -> [_ w4639]
                          tunnel: w4596 -> [_ w4638]
                          tunnel: w4595 -> [_ w4603]
                          tunnel: w4592 -> [_ w4635]
                          tunnel: w4591 -> [_ w4634]
                          tunnel: w4590 -> [_ w4632]
                          tunnel: w4589 -> [_ w4624]
                          frame False {
                          }
                          frame True {
                            n2476 = local read "TDMS LAB05-1"() -> (w4637:refnum<k34>)
                            n2477 = Build Array(w4634) -> (w4629:dbl[])
                            n2478 = Build Array(w4632) -> (w4628:dbl[])
                            n2479 = Build Array(w4639) -> (w4627:dbl[])
                            n2480 = Build Array(w4640) -> (w4626:dbl[])
                            n2481 = Build Array(w4635) -> (w4631:dbl[])
                            n2482 = Build Array(w4633) -> (w4630:dbl[])
                            n2483 = Build Array(w4638) -> (w4625:dbl[])
                            n2484 = Build Array("AMPS ON", "AMPS OFF", "VOLTS", "PF", "TEMP Live", "TEMP Neut", "CYCLE") -> (w4608:string[])
                            n2485 = Bundle By Name("Y"=w4631, "t0"=w4624) -> (w4623:waveform(dbl))  [unwired: 1 in]
                            n2486 = Bundle By Name("Y"=w4630, "t0"=w4624) -> (w4622:waveform(dbl))  [unwired: 1 in]
                            n2487 = Bundle By Name("Y"=w4629, "t0"=w4624) -> (w4621:waveform(dbl))  [unwired: 1 in]
                            n2488 = Bundle By Name("Y"=w4628, "t0"=w4624) -> (w4620:waveform(dbl))  [unwired: 1 in]
                            n2489 = Bundle By Name("Y"=w4627, "t0"=w4624) -> (w4619:waveform(dbl))  [unwired: 1 in]
                            n2490 = Bundle By Name("Y"=w4626, "t0"=w4624) -> (w4618:waveform(dbl))  [unwired: 1 in]
                            n2491 = Bundle By Name("Y"=w4625, "t0"=w4624) -> (w4617:waveform(dbl))  [unwired: 1 in]
                            n2492 = Build Array(w4623, w4622, w4621, w4620, w4619, w4618, w4617) -> (w4616:waveform(dbl)[])
                            n2493 = TDMS Write(0:w4637, 5:"TEST VALUES", 7:w4608, 9:w4616) -> (4:w4607:refnum<k34>, 6:w4606:string, 15:w4605:errorcluster)  [unwired: 2 in, 1 out]
                            n2494 = TDMS Write(0:w4607, 5:w4606, 7:"TIME", 9:w4603, 11:w4605) -> (15:w4602:errorcluster)  [unwired: 1 in, 3 out]
                            n2495 = local write "data file error"(w4602) -> ()
                          }
                        }
                      }
                    }
                  }
                }
              }
              frame #9 {
                n2496 = case shown="True" w4641 {
                  tunnel: w4645 -> [_ w4650]
                  tunnel: w4644 -> [_ w4649]
                  tunnel: w4643 -> [_ w4647]
                  tunnel: w4642 -> [_ w4646]
                  frame False {
                  }
                  frame True {
